vi "Next Step.vi"(8 "error in (no error)":errorcluster, 11 "Magnetic Field Lakeshore Scan in":refnum<class "Magnetic Field Lakeshore Scan.lvclass">) -> (0 "error out":errorcluster, 1 "Current Step":u32, 2 "Current Position":dbl, 3 "Magnetic Field Lakeshore Scan out":refnum<class "Magnetic Field Lakeshore Scan.lvclass">)   [LabVIEW 2023, in "Magnetic Field Lakeshore Scan.lvclass"]
doc: "(Dynamic) Move to the next preconfigured step of this Scanner, and return the current position (actual, not intended) of this Scanner. Increment the step counter by one."
uses:
  Magnetic Field Lakeshore Scan.lvclass
  Scanner/Scanner.lvclass
  Instruments/Utility Classes/Scannable/Scannable.lvclass
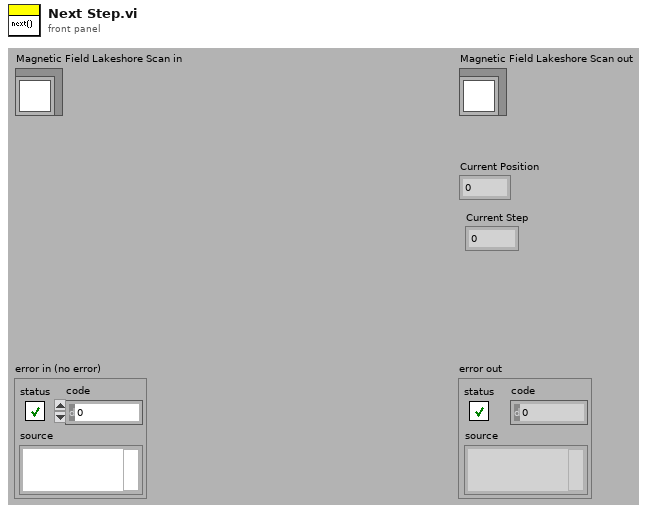
[diagram p1: front panel]
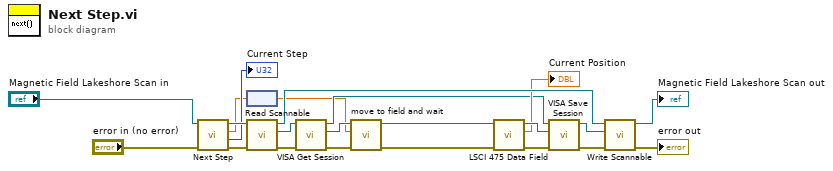
[diagram p0: block diagram]
diagram:
  n1 = call-parent "Next Step.vi"("error in (no error)"="error in (no error)", "Scanner in"="Magnetic Field Lakeshore Scan in") -> ("error out"=w22:errorcluster, "Current Step"=→"Current Step":u32, "Current Position"=w2:dbl, "Scanner out"=w21:refnum<class "Magnetic Field Lakeshore Scan.lvclass">)  [unwired: 6 out]
  n2 = node(w2) -> (w1:dbl[unit])
  n3 = call-dynamic "Read Scannable.vi"("error in (no error)"=w22, "Scanner.lvclass in"=w21) -> ("error out"=w18:errorcluster, "Scannable.lvclass"=w4:refnum<class "Scannable.lvclass">, "Scanner.lvclass out"=w20:refnum<class "Magnetic Field Lakeshore Scan.lvclass">)  [unwired: 7 out]
  n4 = call-dynamic "VISA Get Session.vi"("error in (no error)"=w18, "Instrument.lvclass in"=w4) -> ("error out"=w17:errorcluster, "VISA Resource Name"=w19:refnum<visa-resource-name>, "Instrument.lvclass out"=w3:refnum<class "Scannable.lvclass">)  [unwired: 7 out]
  n5 = call "move to field and wait.vi"("error in (no error)"=w17, "Setpoint"=w1, "VISA session"=w19) -> ("error out"=w12:errorcluster, "dup VISA session"=w14:refnum<visa-resource-name>)  [unwired: 7 in]
  n6 = call "LSCI 475 Data Field.vi"("error in (no error)"=w12, "VISA session"=w14) -> ("error out"=w11:errorcluster, "Field Reading"=→"Current Position":dbl, "dup VISA session"=w13:refnum<visa-resource-name>)  [unwired: 7 in]
  n7 = call-dynamic "VISA Save Session.vi"("error in (no error)"=w11, "VISA Resource Name"=w13, "Instrument.lvclass in"=w3) -> ("error out"=w16:errorcluster, "Instrument.lvclass out"=w15:refnum<class "Scannable.lvclass">)  [unwired: 7 out]
  n8 = call-dynamic "Write Scannable.vi"("error in (no error)"=w16, "Scannable.lvclass"=w15, "Scanner.lvclass in"=w20) -> ("error out"=→"error out":errorcluster, "Scanner.lvclass out"=→"Magnetic Field Lakeshore Scan out":refnum<class "Magnetic Field Lakeshore Scan.lvclass">)  [unwired: 7 out]
